vi "String Array Replace Local Decimal Separators 1D.vi"(1 "array in":string[](array[string])) -> (0 "array out":string[](array[string]))   [LabVIEW 2020]
doc: "This VI takes matrix of strings and tries to replace local decimal separators by dot."
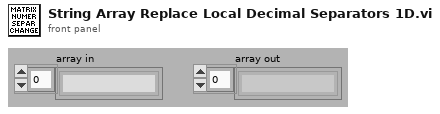
[diagram p1: front panel]
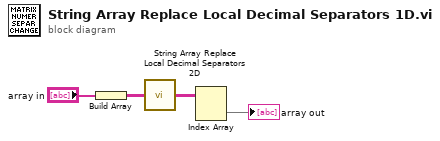
[diagram p0: block diagram]
diagram:
  n1 = Build Array("array in") -> (w3:string[][])
  n2 = call "String Array Replace Local Decimal Separators 2D.vi"("array in"=w3) -> ("array out"=w2:string[][])
  n3 = Index Array(array=w2) -> (element=→"array out":string[])  [unwired: 2 in]
